vi "Configure SSL.vi"(5 "private key file":path, 6 "verify server":bool, 7 "private key password":string, 8 "error in":errorcluster, 9 "client certificate file":path, 10 "CA certificate file":path, 11 "session in":refnum<class "Session.lvclass">) -> (0 "error out":errorcluster, 3 "session out":refnum<class "Session.lvclass">)   [LabVIEW 2019, in "NI_Advanced HTTP Client.lvlib" / "Session.lvclass"]
doc: "Provides Secure Sockets Layer (SSL) authentication for web requests. Use SSL authentication with other HTTP VIs to send web requests to a server, web page, or web service using SSL."
uses:
  Session.lvclass
  Session.lvclass/Session.ctl
  lvwebclient_32.dll
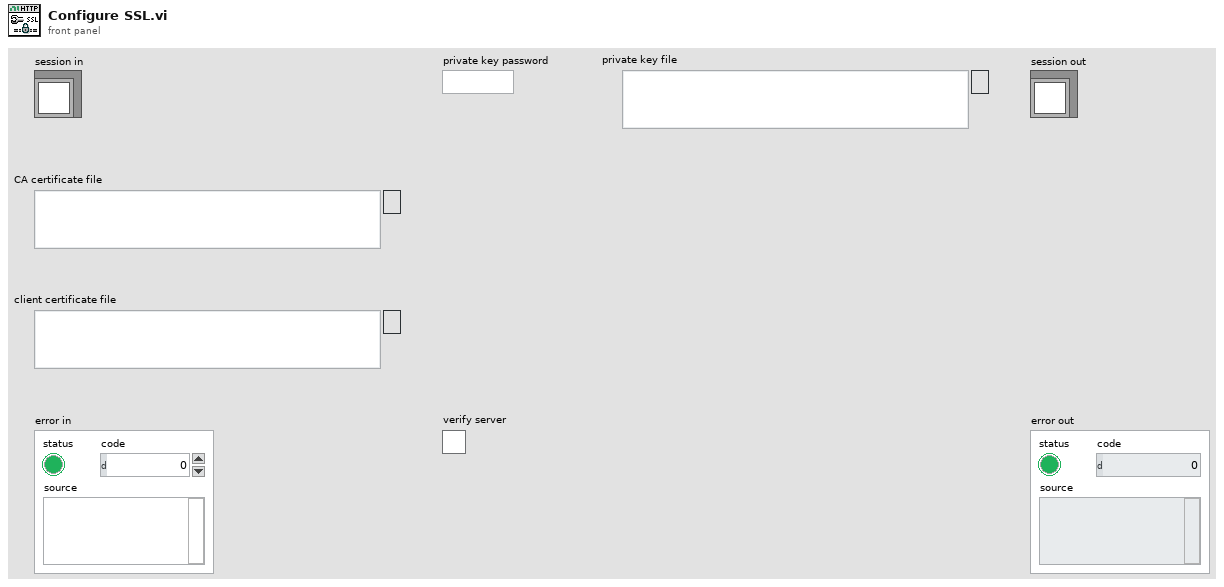
[diagram p1: front panel]
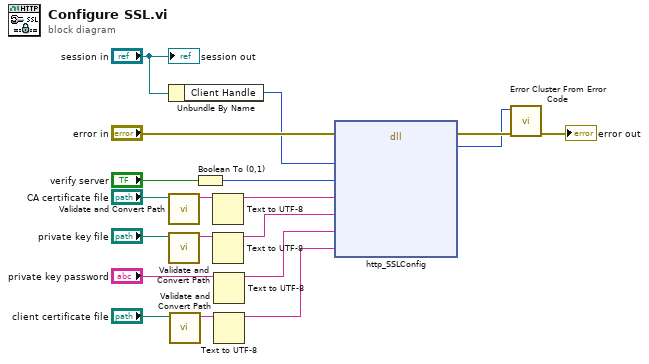
[diagram p0: block diagram]
diagram:
  n1 = Unbundle By Name("session in") -> ("Client Handle"=w13:u32)
  n2 = call "Validate and Convert Path.vi"("path"="CA certificate file") -> ("validated path as string"=w15:string)  [unwired: 10 in]
  n3 = call "Validate and Convert Path.vi"("path"="private key file") -> ("validated path as string"=w7:string)  [unwired: 10 in]
  n4 = call "Validate and Convert Path.vi"("path"="client certificate file") -> ("validated path as string"=w3:string)  [unwired: 10 in]
  n5 = Boolean To (0,1)(Boolean="verify server") -> (0, 1=w12:i16)
  n6 = Text to UTF-8(11:w15) -> (3:w9:string)  [unwired: 2 in, 1 out]
  n7 = Text to UTF-8(11:w7) -> (3:w6:string)  [unwired: 2 in, 1 out]
  n8 = Text to UTF-8(11:"private key password") -> (3:w4:string)  [unwired: 2 in, 1 out]
  n9 = Text to UTF-8(11:w3) -> (3:w1:string)  [unwired: 2 in, 1 out]
  n10 = dll-call lib="C:/source/github/ni-adv-http-api/Advanced HTTP Client/lvwebclient_*.*" fn="http_SSLConfig"(error in="error in", "handle"=w13, "doServerCheck"=w12, "CACertFile"=w9, "privateKeyFile"=w6, "pkPasswd"=w4, "clientCertFile"=w1) -> (error out=w18:errorcluster, "return"=w14:i32)  [unwired: 8 in, 1 out]
  n11 = call <vilib>:"Error Cluster From Error Code.vi"("error in (no error)"=w18, "error code (0)"=w14) -> ("error out"=→"error out":errorcluster)  [unwired: 7 in]
  "session out" <- "session in"
